vi "ReftoDVR--SMO.vi"(10 "Ref":u32 format="%08x") -> (2 "Ref":T1)   [LabVIEW 2019, in "SMO.lvclass"]
doc: "JKI State Machine Objects (SMO) 1.3.0.56\nJKI - JKI\nCopyright (c) 2017, JKI"
uses:
  SMO.lvclass
  Typedefs/PrivateData--Ref.ctl
  Typedefs/PrivateData--Cluster.ctl
  Typedefs/Parent Call--Enum.ctl
  Typedefs/RegisteredProcessData--Cluster.ctl
  Typedefs/Process Error Notification--Cluster.ctl
  Typedefs/Protected Events.ctl
  Typedefs/StopProcessEventData--Cluster.ctl
  Typedefs/AbortProcessEventData--Cluster.ctl
  Typedefs/SMO Dependency Event--Cluster.ctl
  Typedefs/SMO Dependency Event--Enum.ctl
  Typedefs/Public Events.ctl
  Typedefs/SMOState --Enum.ctl
  Typedefs/Reserve State--Enum.ctl
  Typedefs/SMO Dependency--Cluster.ctl
  Support/Attribute/Attribute.lvclass
  Typedefs/Accessibility--Cluster.ctl
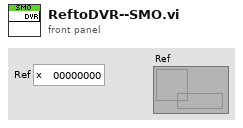
[diagram p1: front panel]
types:
  T1 = typedef "SMO.lvclass/PrivateData--Ref.ctl" = refnum<data-value>
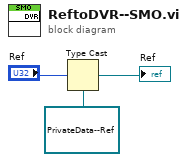
[diagram p0: block diagram]
diagram:
  n1 = Type Cast(type=T1 refnum ("data value reference"), x="Ref") -> (*(type *) &x=→"Ref":T1)
